vi "Ping_Network.vi"(7 "IP/Default Gateway (T/F)":bool, 8 "Error In":errorcluster, 11 "Default Gateway/IP":string="Default Gateway") -> (0 "Error Out":errorcluster, 3 "Terminal Output":string)   [LabVIEW 2017]
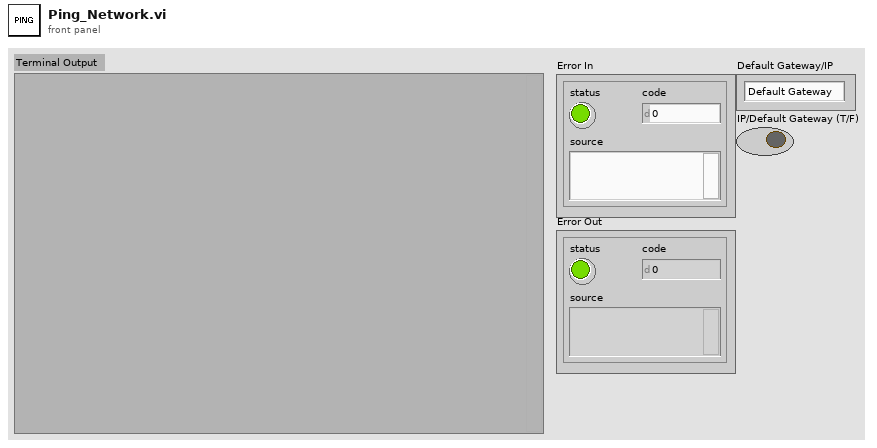
[diagram p1: front panel]
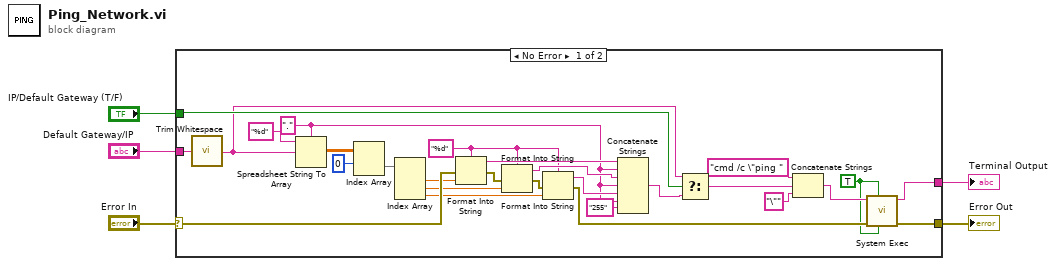
[diagram p0: block diagram]
diagram:
  n1 = case shown="No Error" "Error In" {
    selector: "Error In" -> [w31 w34]
    tunnel: [w33 w34] -> w4
    tunnel: "Default Gateway/IP" -> [w32 _]
    tunnel: [w27 _] -> w2
    tunnel: "IP/Default Gateway (T/F)" -> [w13 _]
    frame No Error {
      w14 = "%d" ("format string")
      w7 = "." ("delimiter (Tab)")
      w9 = TRUE ("wait until completion? (T)")
      n2 = call <vilib>:"Trim Whitespace.vi"("string"=w32) -> ("trimmed string"=w10:string)  [unwired: 1 in]
      n3 = Spreadsheet String To Array(delimiter (Tab)=w7, format string="%d", spreadsheet string=w10) -> (array=w24:dbl[][])  [unwired: 1 in]
      n4 = Index Array(array=w24, index (row)=0) -> (element=w21:dbl[])  [unwired: 1 in]
      n5 = Index Array(array=w21) -> (element #1=w22:dbl, element #2=w18:dbl, element #3=w17:dbl)  [unwired: 3 in]
      n6 = Format Into String(format string=w14, error in=w31, w22) -> (resulting string=w16:string, error out=w20:errorcluster)  [unwired: 1 in]
      n7 = Format Into String(format string=w14, error in=w20, w18) -> (resulting string=w15:string, error out=w19:errorcluster)  [unwired: 1 in]
      n8 = Format Into String(format string=w14, error in=w19, w17) -> (resulting string=w8:string, error out=w26:errorcluster)  [unwired: 1 in]
      n9 = Concatenate Strings(w16, w7, w15, w7, w8, w7, "255" ("string")) -> (w11:string)
      n10 = Select(t=w10, s=w13, f=w11) -> (s? t:f=w12:string)
      n11 = Concatenate Strings("cmd /c \"ping " ("command line"), w12, "\"" ("string")) -> (w30:string)
      n12 = call <vilib>:"System Exec.vi"("run minimized? (F)"=w9, "wait until completion? (T)"=w9, "error in (no error)"=w26, "command line"=w30) -> ("error out"=w33:errorcluster, "standard output"=w27:string)  [unwired: 4 in, 2 out]
    }
    frame Error {
    }
  }
  "Error Out" <- w4
  "Terminal Output" <- w2
